vi "Autonomous Independent.vi"   [LabVIEW 2023]
doc: "This VI is called when autonomous begins, and will automatically be terminated when autonomous ends. You can carry out timed or sensor driven robot movement independently without needing to return to the caller."
uses:
  Arm2/ArmGetSetpointEnum.ctl
  <vilib>/Utility/error.llb/Trim Whitespace One-Sided.vi
  <vilib>/Rock Robotics/Network Tables/NT Read String.vi
panel:
  # "Be sure to right-click and choose Data Operations>>Make Current Value default if you want to save the array values with the VI"
types:
  T1 = typedef "ArmGetSetpointEnum.ctl" = enum16{"ArmFloorPickup", "ArmAmpDeposit", "ArmSpeakerShoot", "ArmStartPosition", "ArmRestPosition", "ArmSourceIntake", "ArmAwayShoot"}
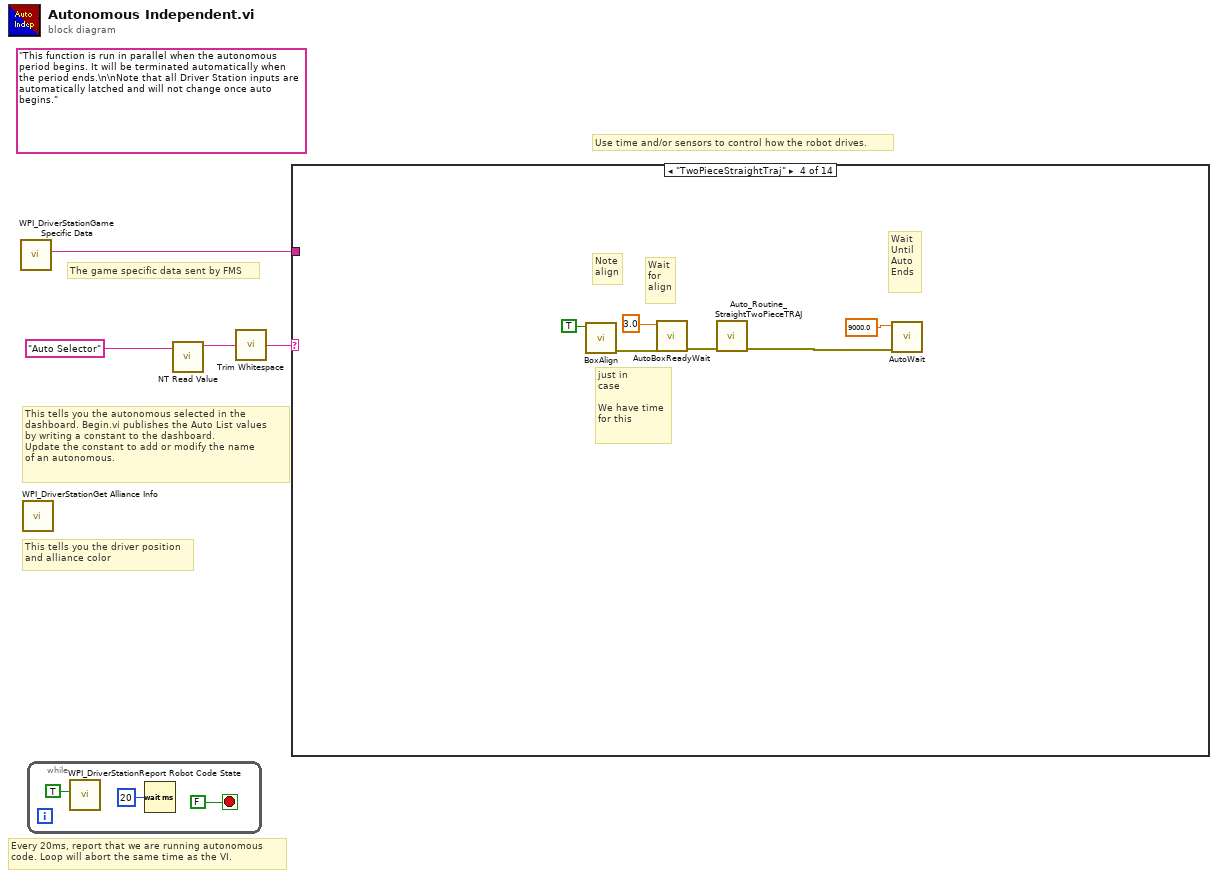
[diagram p0: block diagram]
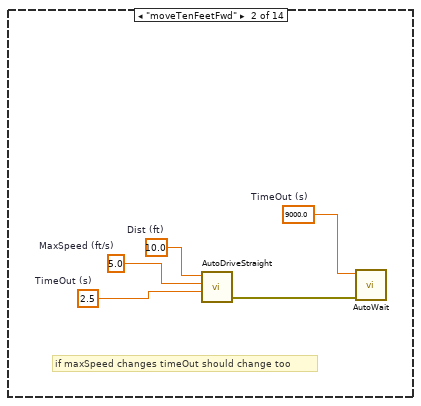
[diagram p3: hidden frame]
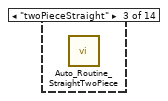
[diagram p4: hidden frame]
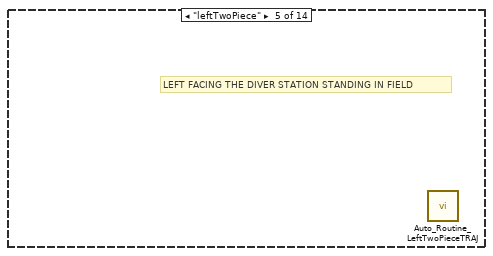
[diagram p5: hidden frame]
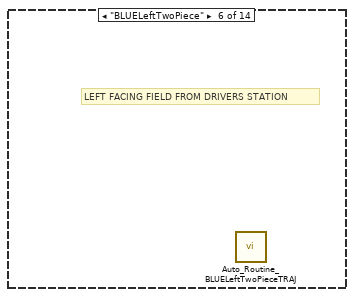
[diagram p6: hidden frame]
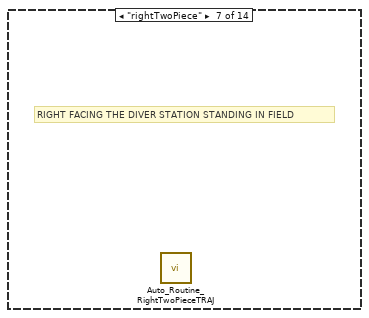
[diagram p7: hidden frame]
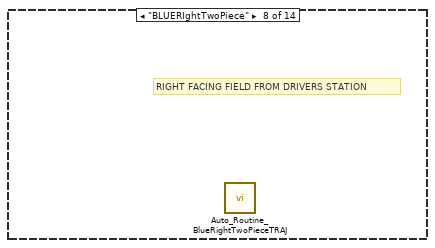
[diagram p8: hidden frame]
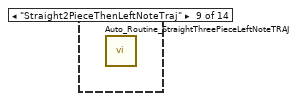
[diagram p9: hidden frame]
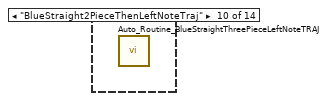
[diagram p10: hidden frame]
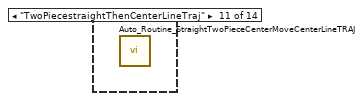
[diagram p11: hidden frame]
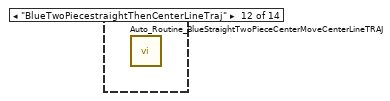
[diagram p12: hidden frame]
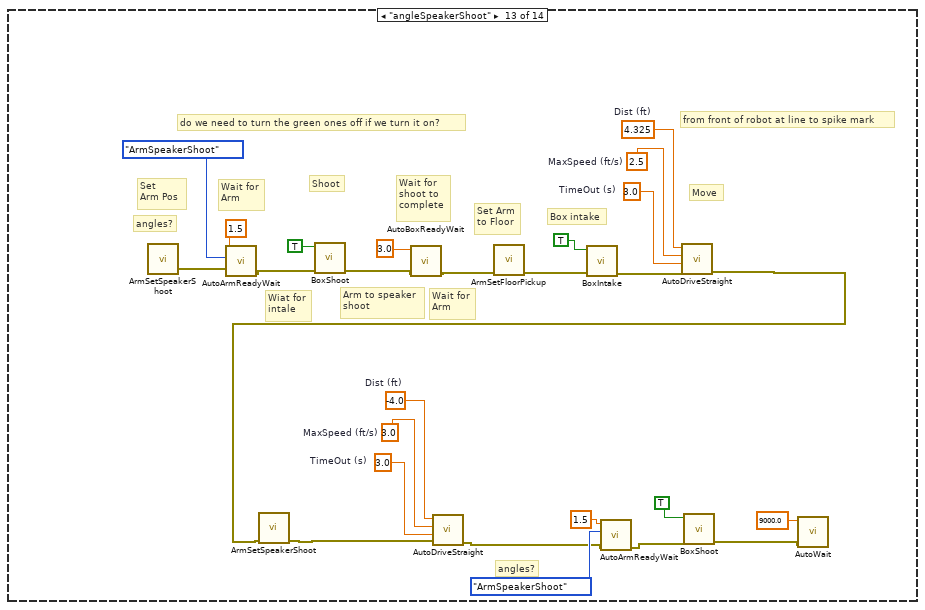
[diagram p13: hidden frame]
diagram:
  (unwired) "This function is run in parallel when the autonomous period begins. It will be terminated automatically when the period ends.\n\nNote that all Driver Station inputs are automatically latched and will not change once auto begins."
  # "The game specific data sent by FMS"
  # "This tells you the autonomous selected in the \ndashboard. Begin.vi publishes the Auto List values\nby writing a constant to the dashboard.\nUpdate the constant to add or modify the name\nof an autonomous."
  # "Every 20ms, report that we are running autonomous\ncode. Loop will abort the same time as the VI."
  # "Use time and/or sensors to control how the robot drives."
  # "This tells you the driver position\nand alliance color"
  n1 = call <vilib>:"WPI_DriverStationGame Specific Data.vi"() -> ("Game Specific Data"=w3:string)  [unwired: 11 in]
  n2 = call <vilib>:"WPI_DriverStationGet Alliance Info.vi"() -> ()  [unwired: 12 out]
  n3 = while {
    stop <- FALSE stop-if-true
    n4 = call <vilib>:"WPI_DriverStationReport Robot Code State.vi"("Autonomous"=TRUE) -> ()  [unwired: 10 in, 1 out]
    n5 = Wait (ms)(milliseconds to wait=u32 20) -> ()  [unwired: 1 out]
  }
  n6 = call-poly <vilib>:"NT Read Value.vi"("name"="Auto Selector" ("Name")) -> ("value"=w1:string)  [unwired: 8 in, 2 out]
  n7 = call <vilib>:"Trim Whitespace.vi"("string"=w1) -> ("trimmed string"=w2:string)  [unwired: 1 in]
  n8 = case shown="\"TwoPieceStraightTraj\"" w2 {
    tunnel: w3 -> [_ _ _ _ _ _ _ _ _ _ _ _ _ _]
    frame Default {
      # "You can put your main auto here, or you can right-click on the case and make any\nother frame be the default case."
      # "This is the frame that will execute if no selection is made, or if it is not recognized"
    }
    frame "moveTenFeetFwd" {
      w8 = 9000.0  # TimeOut (s)
      w10 = 2.5  # TimeOut (s)
      w11 = 5.0  # MaxSpeed (ft/s)
      w12 = 10.0  # Dist (ft)
      # "if maxSpeed changes timeOut should change too"
      n9 = call "AutoDriveStraight.vi"("TimeOut (s)"=w10, "MaxSpeed (ft/s)"=w11, "Dist (ft)"=w12) -> ("error out"=w9:errorcluster)  [unwired: 8 in]
      n10 = call "AutoWait.vi"("error in (no error)"=w9, "TimeOut (s)"=w8) -> ()  [unwired: 9 in, 1 out]
    }
    frame "twoPieceStraight" {
      n11 = call "Auto_Routine_StraightTwoPiece.vi"() -> ()  [unwired: 11 in, 1 out]
    }
    frame "TwoPieceStraightTraj" {
      # "just in\ncase\n\nWe have time\nfor this"
      # "Wait\nfor\nalign"
      # "Note\nalign"
      # "Wait\nUntil\nAuto \nEnds"
      n12 = call "BoxAlign.vi"("box align"=TRUE) -> ("error out"=w14:errorcluster)  [unwired: 10 in]
      n13 = call "AutoBoxReadyWait.vi"("error in (no error)"=w14, "TimeOut (s)"=3.0) -> ("error out"=w13:errorcluster)  [unwired: 9 in]
      n14 = call "Auto_Routine_StraightTwoPieceTRAJ.vi"("error in (no error)"=w13) -> ("error out"=w17:errorcluster)  [unwired: 10 in]
      n15 = call "AutoWait.vi"("error in (no error)"=w17, "TimeOut (s)"=9000.0) -> ()  [unwired: 9 in, 1 out]
    }
    frame "leftTwoPiece" {
      # "LEFT FACING THE DIVER STATION STANDING IN FIELD"
      n16 = call "Auto_Routine_LeftTwoPieceTRAJ.vi"() -> ()  [unwired: 12 in]
    }
    frame "BLUELeftTwoPiece" {
      # "LEFT FACING FIELD FROM DRIVERS STATION"
      n17 = call "Auto_Routine_BLUELeftTwoPieceTRAJ.vi"() -> ()  [unwired: 12 in]
    }
    frame "rightTwoPiece" {
      # "RIGHT FACING THE DIVER STATION STANDING IN FIELD"
      n18 = call "Auto_Routine_RightTwoPieceTRAJ.vi"() -> ()  [unwired: 12 in]
    }
    frame "BLUERIghtTwoPiece" {
      # "RIGHT FACING FIELD FROM DRIVERS STATION"
      n19 = call "Auto_Routine_BlueRightTwoPieceTRAJ.vi"() -> ()  [unwired: 12 in]
    }
    frame "Straight2PieceThenLeftNoteTraj" {
      n20 = call "Auto_Routine_StraightThreePieceLeftNoteTRAJ.vi"() -> ()  [unwired: 11 in, 1 out]
    }
    frame "BlueStraight2PieceThenLeftNoteTraj" {
      n21 = call "Auto_Routine_BlueStraightThreePieceLeftNoteTRAJ.vi"() -> ()  [unwired: 11 in, 1 out]
    }
    frame "TwoPiecestraightThenCenterLineTraj" {
      n22 = call "Auto_Routine_StraightTwoPieceCenterMoveCenterLineTRAJ.vi"() -> ()  [unwired: 11 in, 1 out]
    }
    frame "BlueTwoPiecestraightThenCenterLineTraj" {
      n23 = call "Auto_Routine_BlueStraightTwoPieceCenterMoveCenterLineTRAJ.vi"() -> ()  [unwired: 11 in, 1 out]
    }
    frame "angleSpeakerShoot" {
      w22 = 3.0  # TimeOut (s)
      w23 = 3.0  # MaxSpeed (ft/s)
      w24 = -4.0  # Dist (ft)
      w41 = 3.0  # TimeOut (s)
      w42 = 2.5  # MaxSpeed (ft/s)
      w43 = 4.325  # Dist (ft)
      # "Wait for\nArm"
      # "Arm to speaker\nshoot"
      # "Wiat for\nintale"
      # "Box intake"
      # "Move"
      # "Set Arm\nto Floor"
      # "Wait for\nshoot to\ncomplete"
      # "Shoot"
      # "Wait for\nArm"
      # "Set\nArm Pos"
      # "do we need to turn the green ones off if we turn it on?"
      # "angles?"
      # "angles?"
      # "from front of robot at line to spike mark"
      n24 = call "ArmSetSpeakerShoot.vi"() -> ("error out"=w34:errorcluster)  [unwired: 11 in]
      n25 = call "AutoArmReadyWait.vi"("error in (no error)"=w34, "ArmSetpoints"=ArmGetSetpointEnum."ArmSpeakerShoot", "TimeOut (s)"=1.5) -> ("error out"=w33:errorcluster)  [unwired: 8 in]
      n26 = call "BoxShoot.vi"("error in (no error)"=w33, "Box shoot"=TRUE) -> ("error out"=w31:errorcluster)  [unwired: 9 in]
      n27 = call "AutoBoxReadyWait.vi"("error in (no error)"=w31, "TimeOut (s)"=3.0) -> ("error out"=w30:errorcluster)  [unwired: 9 in]
      n28 = call "ArmSetFloorPickup.vi"("error in (no error)"=w30) -> ("error out"=w36:errorcluster)  [unwired: 10 in]
      n29 = call "BoxIntake.vi"("error in (no error)"=w36, "Box intake"=TRUE) -> ("error out"=w35:errorcluster)  [unwired: 9 in]
      n30 = call "AutoDriveStraight.vi"("error in (no error)"=w35, "TimeOut (s)"=w41, "MaxSpeed (ft/s)"=w42, "Dist (ft)"=w43) -> ("error out"=w20:errorcluster)  [unwired: 7 in]
      n31 = call "ArmSetSpeakerShoot.vi"("error in (no error)"=w20) -> ("error out"=w19:errorcluster)  [unwired: 10 in]
      n32 = call "AutoDriveStraight.vi"("error in (no error)"=w19, "TimeOut (s)"=w22, "MaxSpeed (ft/s)"=w23, "Dist (ft)"=w24) -> ("error out"=w21:errorcluster)  [unwired: 7 in]
      n33 = call "AutoArmReadyWait.vi"("error in (no error)"=w21, "ArmSetpoints"=ArmGetSetpointEnum."ArmSpeakerShoot", "TimeOut (s)"=1.5) -> ("error out"=w28:errorcluster)  [unwired: 8 in]
      n34 = call "BoxShoot.vi"("error in (no error)"=w28, "Box shoot"=TRUE) -> ("error out"=w38:errorcluster)  [unwired: 9 in]
      n35 = call "AutoWait.vi"("error in (no error)"=w38, "TimeOut (s)"=9000.0) -> ()  [unwired: 9 in, 1 out]
    }
    frame "Your Turn" {
    }
  }
